vi "connectionStatus.vi"(8 "error in (no error)":errorcluster, 10 "status":string, 11 "TcpServerTel in":refnum<class "TcpServerTel.lvclass">) -> (0 "error out":errorcluster, 3 "TcpServerTel out":refnum<class "TcpServerTel.lvclass">)   [LabVIEW 2018, in "TcpServerTel.lvclass"]
doc: "Send a generic user event to inform the tcpServerTel status."
uses:
  TcpServerTel.lvclass
  home/pcortes/github/ts_labview_tcp_json/src/TcpServerBase/TcpServerBase.lvclass
  TcpServerBase/TcpServerBase.lvclass/TcpServerBase.ctl
  TcpServerBase/TcpServerBase.lvclass
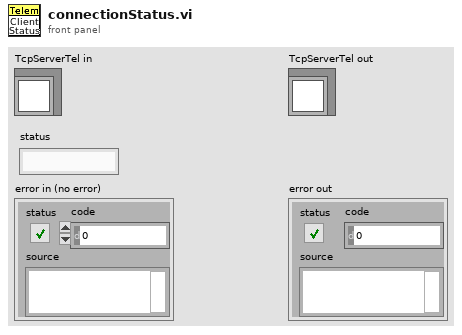
[diagram p1: front panel]
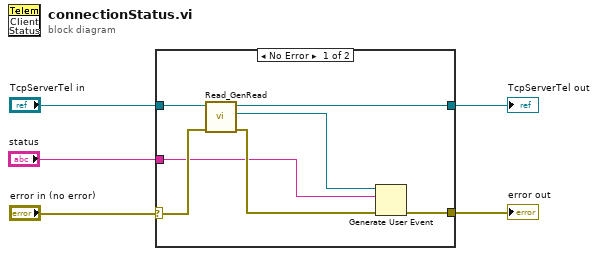
[diagram p0: block diagram]
diagram:
  n1 = case shown="No Error" "error in (no error)" {
    selector: "error in (no error)" -> [w10 w14]
    tunnel: [w12 w14] -> w5
    tunnel: [w9 w13] -> w3
    tunnel: "TcpServerTel in" -> [w8 w13]
    tunnel: "status" -> [w7 _]
    frame No Error {
      n2 = call "Read_GenRead.vi"("error in (no error)"=w10, "TcpServerBase in"=w8) -> ("error out"=w11:errorcluster, "GenRead"=w6:refnum<user-event>, "TcpServerBase out"=w9:refnum<class "TcpServerTel.lvclass">)  [unwired: 7 in]
      n3 = Generate User Event(user event=w6, event data cluster=w7, error in=w11) -> (error out=w12:errorcluster)  [unwired: 1 in, 1 out]
    }
    frame Error {
    }
  }
  "error out" <- w5
  "TcpServerTel out" <- w3
